vi "Enum Counts.vi"(10 "Enum In":i64=32000000000 format="%.0p") -> (2 "Counts Out":i64)   [LabVIEW 2024]
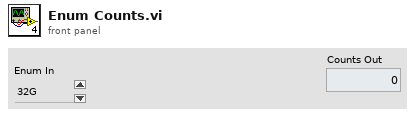
[diagram p1: front panel]
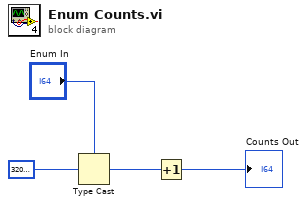
[diagram p0: block diagram]
diagram:
  n1 = Type Cast(type="Enum In", x=i64 32000000000) -> (*(type *) &x=w1:i64)
  n2 = Increment(x=w1) -> (x+1=→"Counts Out":i64)
